vi "OmniDrive.vi"() -> ()   [LabVIEW 2014]
uses:
  <vilib>/Rock Robotics/WPI/RobotDrive/WPI_RobotDriveDevRef.ctl
  <vilib>/Rock Robotics/WPI/MotorControl/WPI_MotorControlDeviceRef.ctl
  <vilib>/Rock Robotics/WPI/MotorControl/WPI_MotorControlType.ctl
  <vilib>/Rock Robotics/SystemInterfaces/Typedef/FPGA_TypedefDigitalModule.ctl
  <vilib>/Rock Robotics/SystemInterfaces/DIO/FPGA_DIOPWMChannel.ctl
  <vilib>/Rock Robotics/WPI/PWM/WPI_PWMDeadband.ctl
  <vilib>/Rock Robotics/WPI/CAN/Jaguar/SubVIs/WPI_CANJaguar_ControlMode.ctl
  <vilib>/Rock Robotics/WPI/CAN/TalonSRX/WPI_CANTalonSRX_APIControlMode.ctl
  <vilib>/Rock Robotics/WPI/PWM/WPI_PWMTransform_ConPane.ctl
  <vilib>/Rock Robotics/SystemInterfaces/NetworkCommunication/NetComm_UsageReport_ResourceType.ctl
panel:
  out "Motor Values":dbl[](array[numeric])
  in  "RobotDriveDevRef":T1={"DevStatus"={"status"=FALSE, "code"=0, "source"=""}, "Motors[]"=[], "Square Inputs"=FALSE, "Max Output"=1.0}
  in  "error in (no error)":errorcluster
  out "error out":errorcluster
  out "RobotDriveDevRef 2":T1={"DevStatus"={"status"=FALSE, "code"=0, "source"=""}, "Motors[]"=[], "Square Inputs"=FALSE, "Max Output"=1.0}
  in  "X axis value":dbl
  in  "Y axis value":dbl
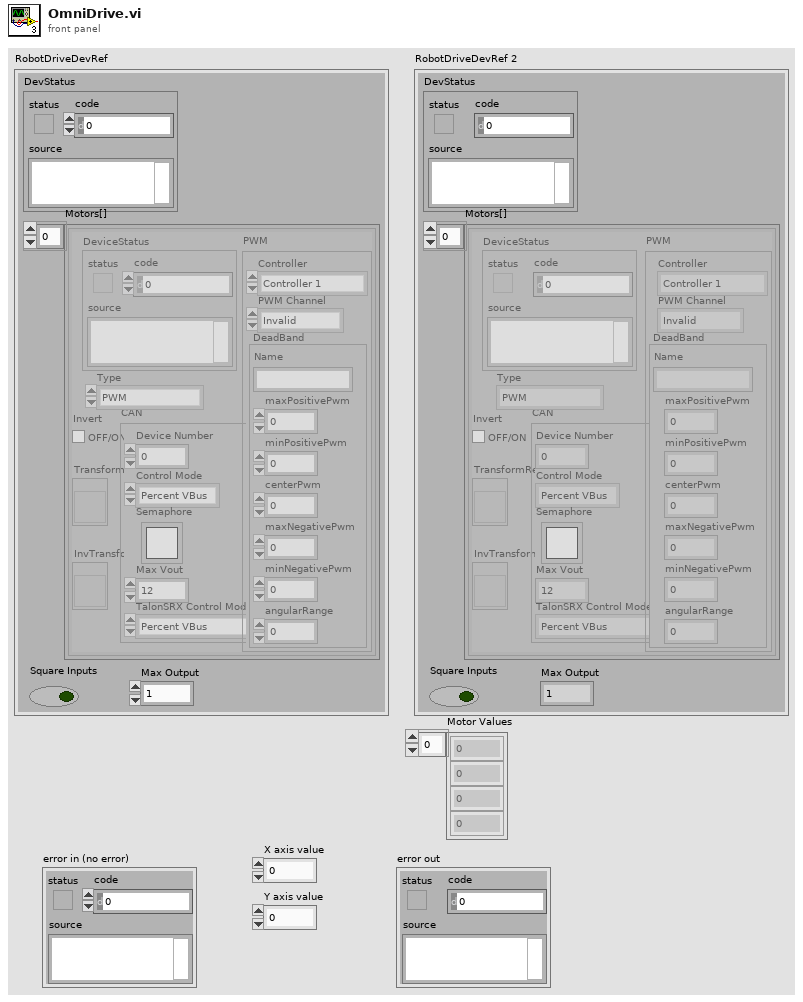
[diagram p1: front panel]
types:
  T1 = typedef "WPI_RobotDriveDevRef.ctl" = cluster{"DevStatus":errorcluster, "Motors[]":T2[], "Square Inputs":bool, "Max Output":dbl}
  T2 = typedef "WPI_MotorControlDeviceRef.ctl" = cluster{"DeviceStatus":errorcluster, "Type":T3, "PWM":cluster{"Controller":T4, "PWM Channel":T5, "DeadBand":T6}, "CAN":cluster{"Device Number":u8, "Control Mode":T7, "Semaphore":T8, "Max Vout":dbl, "TalonSRX Control Mode":T9}, "Invert":bool, "TransformRef":T10, "InvTransformRef":T10}
  T3 = typedef "WPI_MotorControlType.ctl" = enum16{"PWM", "CAN", "CANTalonSRX"}
  T4 = typedef "FPGA_TypedefDigitalModule.ctl" = enum16{"Controller 1"}
  T5 = typedef "FPGA_DIOPWMChannel.ctl" = enum8{"PWM 0", "PWM 1", "PWM 2", "PWM 3", "PWM 4", "PWM 5", "PWM 6", "PWM 7", "PWM 8", "PWM 9", "PWM MXP 0", "PWM MXP 1", "PWM MXP 2", "PWM MXP 3", "PWM MXP 4", "PWM MXP 5", "PWM MXP 6", "PWM MXP 7", "PWM MXP 8", "PWM MXP 9", "Invalid"}
  T6 = typedef "WPI_PWMDeadband.ctl" = cluster{"Name":string, "maxPositivePwm":i32, "minPositivePwm":i32, "centerPwm":i32, "maxNegativePwm":i32, "minNegativePwm":i32, "angularRange":u16}
  T7 = typedef "WPI_CANJaguar_ControlMode.ctl" = enum8{"Percent VBus", "Current", "Speed", "Position", "Voltage"}
  T8 = typedef "Semaphore RefNum" = refnum<k1>
  T9 = typedef "WPI_CANTalonSRX_APIControlMode.ctl" = enum8{"Percent VBus", "Speed", "Position", "Slave", "Unchanged / Invalid"}
  T10 = typedef "WPI_PWMTransform_ConPane.ctl" = refnum<vi>
  T11 = typedef "NetComm_UsageReport_ResourceType.ctl" = enum8{"Controller", "Module", "Language", "CANPlugin", "Accelerometer", "ADXL345", "AnalogChannel", "AnalogTrigger", "AnalogTriggerOutput", "CANJaguar", "Compressor", "Counter", "Dashboard", "DigitalInput", "DigitalOutput", "DriverStationCIO", "DriverStationEIO", "DriverStationLCD", "Encoder", "GearTooth", "Gyro", "I2C", "Framework", "Jaguar", "Joystick", "Kinect", "KinectStick", "PIDController", "Preferences", "PWM", "Relay", "RobotDrive", "SerialPort", "Servo", "Solenoid", "SPI", "Task", "Ultrasonic", "Victor", "Button", "Command", "AxisCamera", "PCVideoServer", "SmartDashboard", "Talon", "HiTechnicColorSensor", "HiTechnicAccel", "HiTechnicCompass", "SRF08", "AnalogOutput", "Victor SP", "Talon SRX", "CAN Talon SRX"}
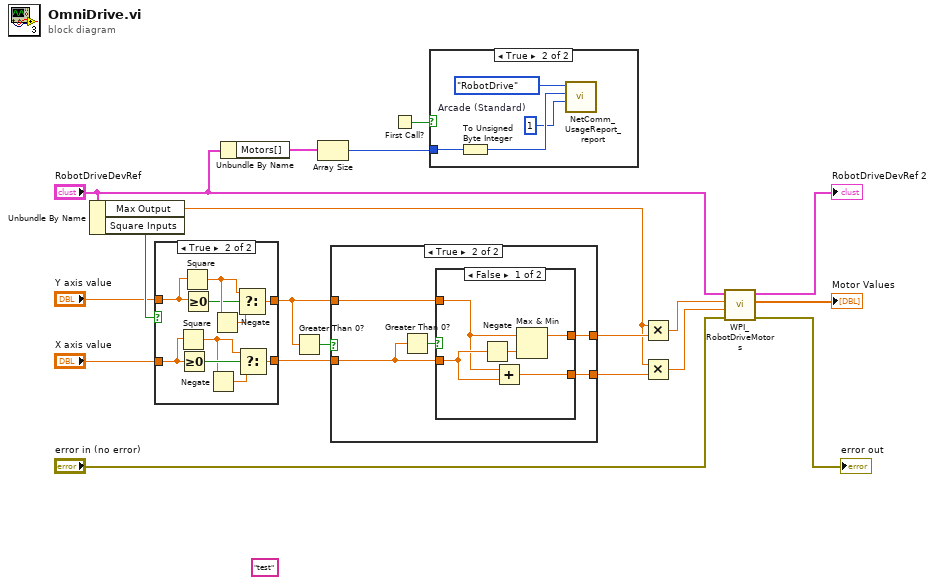
[diagram p0: block diagram]
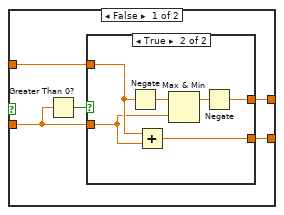
[diagram p3: hidden frame]
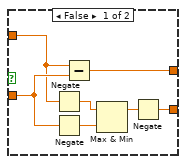
[diagram p4: hidden frame]
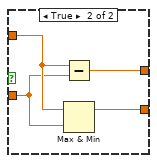
[diagram p5: hidden frame]
diagram:
  (unwired) "test"
  n1 = Unbundle By Name("RobotDriveDevRef") -> ("Max Output"=w8:dbl, "Square Inputs"=w18:bool)
  n2 = case shown="True" w18 {
    tunnel: [w20 w31] -> w15
    tunnel: [w21 w30] -> w16
    tunnel: "X axis value" -> [w20 w29]
    tunnel: "Y axis value" -> [w21 w28]
    frame False {
    }
    frame True {
      n3 = Square(x=w29) -> (x^2=w26:dbl)
      n4 = Greater Or Equal To 0?(x=w29) -> (x >= 0?=w27:bool)
      n5 = Square(x=w28) -> (x^2=w23:dbl)
      n6 = Greater Or Equal To 0?(x=w28) -> (x >= 0?=w22:bool)
      n7 = Negate(x=w26) -> (-x=w25:dbl)
      n8 = Negate(x=w23) -> (-x=w24:dbl)
      n9 = Select(t=w23, s=w22, f=w24) -> (s? t:f=w30:dbl)
      n10 = Select(t=w26, s=w27, f=w25) -> (s? t:f=w31:dbl)
    }
  }
  n11 = Unbundle By Name("RobotDriveDevRef") -> ("Motors[]"=w3:T2[])
  n12 = Greater Than 0?(x=w16) -> (x > 0?=w17:bool)
  n13 = Array Size(array=w3) -> (size(s)=w2:i32)
  n14 = case shown="True" w17 {
    tunnel: w15 -> [w35 w53]
    tunnel: w16 -> [w34 w52]
    tunnel: [w33 w51] -> w14
    tunnel: [w32 w50] -> w10
    frame False {
      n15 = Greater Than 0?(x=w35) -> (x > 0?=w36:bool)
      n16 = case shown="True" w36 {
        tunnel: w35 -> [w43 w45]
        tunnel: w34 -> [w41 w46]
        tunnel: [w37 w47] -> w33
        tunnel: [w38 w44] -> w32
        frame False {
          n17 = Negate(x=w41) -> (-x=w42:dbl)
          n18 = Negate(x=w43) -> (-x=w40:dbl)
          n19 = Subtract(x=w41, y=w43) -> (x-y=w37:dbl)
          n20 = Max & Min(x=w42, y=w40) -> (max(x,y)=w39:dbl)  [unwired: 1 out]
          n21 = Negate(x=w39) -> (-x=w38:dbl)
        }
        frame True {
          n22 = Negate(x=w46) -> (-x=w49:dbl)
          n23 = Add(x=w46, y=w45) -> (x+y=w44:dbl)
          n24 = Max & Min(x=w49, y=w45) -> (max(x,y)=w48:dbl)  [unwired: 1 out]
          n25 = Negate(x=w48) -> (-x=w47:dbl)
        }
      }
    }
    frame True {
      n26 = Greater Than 0?(x=w53) -> (x > 0?=w54:bool)
      n27 = case shown="False" w54 {
        tunnel: w53 -> [w59 w61]
        tunnel: w52 -> [w56 w62]
        tunnel: [w57 w60] -> w51
        tunnel: [w55 w63] -> w50
        frame False {
          n28 = Negate(x=w59) -> (-x=w58:dbl)
          n29 = Add(x=w56, y=w59) -> (x+y=w55:dbl)
          n30 = Max & Min(x=w56, y=w58) -> (max(x,y)=w57:dbl)  [unwired: 1 out]
        }
        frame True {
          n31 = Subtract(x=w62, y=w61) -> (x-y=w60:dbl)
          n32 = Max & Min(x=w62, y=w61) -> (max(x,y)=w63:dbl)  [unwired: 1 out]
        }
      }
    }
  }
  n33 = First Call?() -> (First Call?: T/F=w5:bool)
  n34 = case shown="True" w5 {
    tunnel: w2 -> [_ w66]
    frame False {
    }
    frame True {
      w64 = u8 1  # Arcade (Standard)
      n35 = To Unsigned Byte Integer(number=w66) -> (unsigned 8bit integer=w65:u8)
      n36 = call <vilib>:"NetComm_UsageReport_report.vi"("Context"=w64, "Instance Number"=w65, "Resource Type"=NetComm_UsageReport_ResourceType."RobotDrive") -> ()  [unwired: 9 in]
    }
  }
  n37 = Multiply(x=w8, y=w14) -> (x*y=w11:dbl)
  n38 = Multiply(x=w8, y=w10) -> (x*y=w9:dbl)
  n39 = call <vilib>:"WPI_RobotDriveMotors.vi"("error in (no error)"="error in (no error)", "RightSpeed"=w9, "LeftSpeed"=w11, "RobotDriveDevRef"="RobotDriveDevRef") -> ("error out"=→"error out":errorcluster, "Motor Values"=→"Motor Values":dbl[], "RobotDriveDevRef"=→"RobotDriveDevRef 2":T1)  [unwired: 5 out]
